vi "期末專題.vi"() -> ()   [LabVIEW 2014]
uses:
  <vilib>/MakerHub/LINX/LMH-LINX.lvlib
  <vilib>/MakerHub/LINX/Public/Peripherals/Digital/Digital Write 1 Chan.vi
  <vilib>/MakerHub/LINX/Public/Peripherals/Digital/Digital Read 1 Chan.vi
  <vilib>/MakerHub/LINX/Public/Utilities/Open Serial.vi
panel:
  out "Waveform Chart":i16[](graph)
  out "訊號開關":bool
  in  "連接通道口":refnum<visa-resource-name>="N/A"
  in  "stop 2":bool
  in  "訊號輸出通道":u8
  in  "訊號輸入通道":u8
  out "今天日期":string="今天日期"
  out "現在時間":string
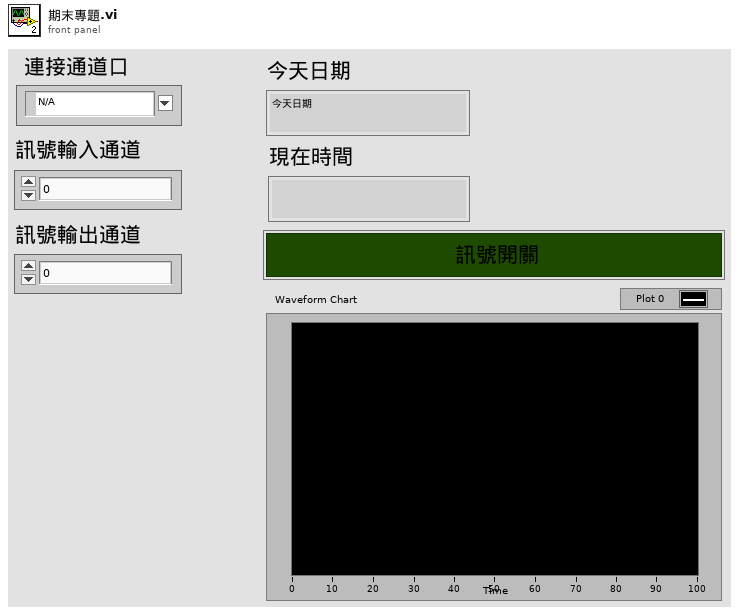
[diagram p1: front panel]
types:
  T1 = typedef "LMH-LINX.lvlib/LINX Ref.ctl" = cluster{"IO":T2, "Interface":T3, "LINX Device Config":T4}
  T2 = typedef "LMH-LINX.lvlib/Platform.ctl" = enum16{"Remote", "Local"}
  T3 = typedef "LMH-LINX.lvlib/Interface.ctl" = enum16{"Serial", "TCP"}
  T4 = typedef "LMH-LINX.lvlib/Device.lvlib/LINX Device Config.ctl" = cluster{"Interface":T3, "COM Port":refnum<visa-resource-name>, "TCP Configuration":T5, "Device Family":u8, "Device ID":u8, "Device Name":string, "TCP Ref":refnum<k5>, "Channels":T6}
  T5 = typedef "LMH-LINX.lvlib/Device.lvlib/TCP Config.ctl" = cluster{"IP Address":string, "Port":u16}
  T6 = typedef "LMH-LINX.lvlib/Channels.ctl" = cluster{"DI":u8[], "DO":u8[], "AI":u8[], "AO":u8[], "PWM":u8[], "QE":u8[], "UART":u8[], "I2C 2":u8[], "SPI":u8[], "CAN":u8[], "Servo":u8[], "AI Ref (V)":dbl, "AI Resolution (Bits)":u8, "AO Ref (V)":dbl, "AO Resolution (Bits)":u8}
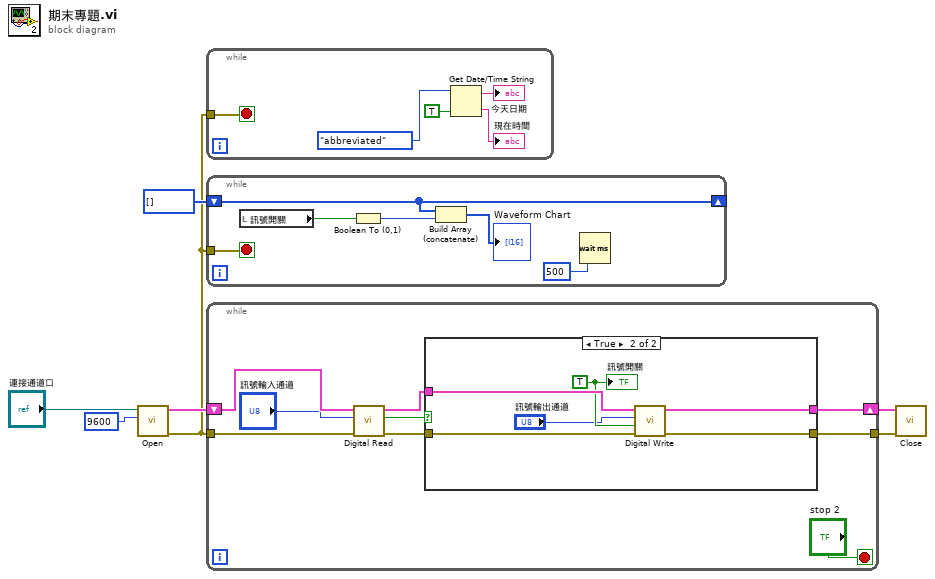
[diagram p0: block diagram]
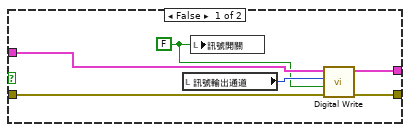
[diagram p2: hidden frame]
diagram:
  n1 = call-poly <vilib>:"Open.vi"("Baud Rate Override"=u32 9600, "Serial Port"="連接通道口") -> ("Error Out"=w1:errorcluster, "LINX Resource"=w6:T1)  [unwired: 7 in, 1 out]
  n2 = while {
    tunnel: w1 -> [w8]
    stop <- w8 stop-if-true
    n3 = Get Date/Time String(date format (0)=enum16{"short", "long", "abbreviated"}."abbreviated", want seconds? (F)=TRUE) -> (date string=→"今天日期":string, time string=→"現在時間":string)  [unwired: 1 in]
  }
  n4 = while {
    shift-right: [w14] -> _
    shift-left: i16[] [] -> [w14]
    tunnel: w1 -> [w16]
    stop <- w16 stop-if-true
    n5 = local read "訊號開關"() -> (w18:bool)
    n6 = Boolean To (0,1)(Boolean=w18) -> (0, 1=w17:i16)
    n7 = Build Array (concatenate)(w14, w17) -> (→"Waveform Chart":i16[])
    n8 = Wait (ms)(milliseconds to wait=u32 500) -> ()  [unwired: 1 out]
  }
  n9 = while {
    shift-right: [w26] -> w4
    shift-left: w6 -> [w27]
    tunnel: w1 -> [w25]
    tunnel: [w24] -> w3
    stop <- "stop 2" stop-if-true
    n10 = call-poly <vilib>:"Digital Read.vi"("Error In"=w25, "DI Channel"="訊號輸入通道", "LINX Resource"=w27) -> ("Error Out"=w21:errorcluster, "DI Value"=w20:bool, "LINX Resource"=w22:T1)  [unwired: 6 in]
    n11 = case shown="True" w20 {
      tunnel: w22 -> [w32 w39]
      tunnel: [w31 w38] -> w26
      tunnel: w21 -> [w30 w37]
      tunnel: [w29 w36] -> w24
      frame False {
        w28 = FALSE
        n12 = local read "訊號輸出通道"() -> (w33:u8)
        n13 = local write "訊號開關"(w28) -> ()
        n14 = call-poly <vilib>:"Digital Write.vi"("Error In"=w30, "Output Value"=w28, "DO Channel"=w33, "LINX Resource"=w32) -> ("Error Out"=w29:errorcluster, "LINX Resource"=w31:T1)  [unwired: 6 in]
      }
      frame True {
        w35 = TRUE
        n15 = call-poly <vilib>:"Digital Write.vi"("Error In"=w37, "Output Value"=w35, "DO Channel"="訊號輸出通道", "LINX Resource"=w39) -> ("Error Out"=w36:errorcluster, "LINX Resource"=w38:T1)  [unwired: 6 in]
        "訊號開關" <- w35
      }
    }
  }
  n16 = call <vilib>:"Close.vi"("Error In"=w3, "LINX Resource"=w4) -> ()  [unwired: 9 in, 1 out]
